vi "Open RS422A.vi"(4 "Source (\"\")":string, 6 "Timeout (25000)":u32=25000, 8 "error in (no error)":errorcluster, 10 "Address (1)":i32=1 min=1 max=99 step=1, 11 "VISA resource name":refnum<visa-resource-name>) -> (0 "error out":errorcluster, 3 "VISA resource name out":refnum<visa-resource-name>)   [LabVIEW 2020, in "Yokogawa GX Series.lvlib"]
doc: "Opens RS-422A/485."
uses:
  <instrlib>/Yokogawa GX Series/Yokogawa GX Series.lvlib
panel:
  # "msec"
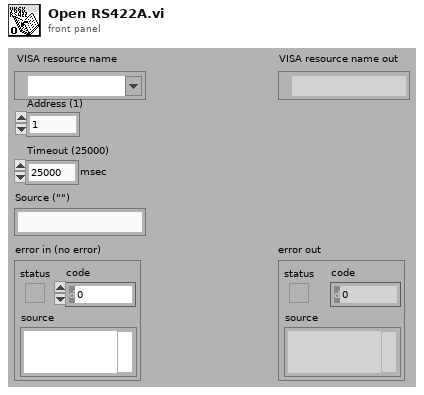
[diagram p1: front panel]
types:
  T1 = cluster{"User Name":string, "User ID":string, "Password":string, "Serial Auth Type (0: Not Auth)":u16, "SMARTDAC+ Type (0: Unknown)":u16, "Bluetooth Password":string}
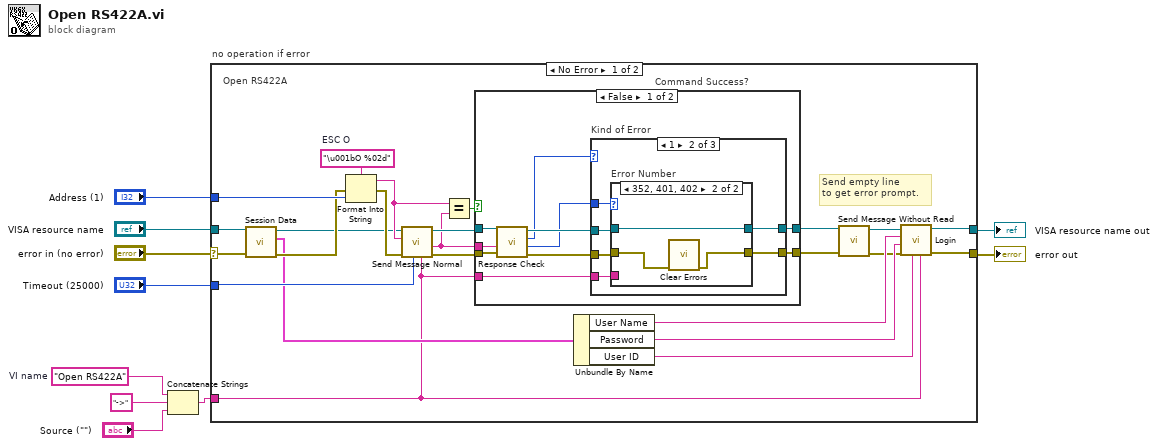
[diagram p0: block diagram]
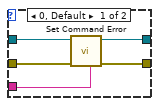
[diagram p3: hidden frame]
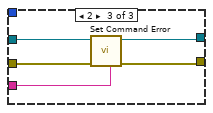
[diagram p4: hidden frame]
diagram:
  w4 = "Open RS422A"  # VI name
  n1 = Concatenate Strings(w4, "->", "Source (\"\")") -> (w2:string)
  n2 = case "no operation if error" shown="No Error" "error in (no error)" {
    selector: "error in (no error)" -> [w18 w68]
    tunnel: "Address (1)" -> [w34 _]
    tunnel: "VISA resource name" -> [w19 w69]
    tunnel: [w23 w69] -> w8
    tunnel: [w22 w68] -> w7
    tunnel: "Timeout (25000)" -> [w28 _]
    tunnel: w2 -> [w11 _]
    frame No Error {
      w33 = "\u001bO %02d"  # ESC O
      # "Send empty line\nto get error prompt."
      # "Open RS422A"
      n3 = call <instrlib>:"Session Data.vi"("error in (no error)"=w18, "VISA resource name"=w19) -> ("error out"=w17:errorcluster, "User Data Out"=w15:T1, "VISA resource name out"=w16:refnum<visa-resource-name>)  [unwired: 7 in]
      n4 = Format Into String(format string=w33, error in=w17, w34) -> (resulting string=w27:string, error out=w29:errorcluster)  [unwired: 1 in]
      n5 = call <instrlib>:"Send Message Normal.vi"("Source (\"\")"=w11, "Timeout (25000)"=w28, "error in (no error)"=w29, "Send Message (\"\")"=w27, "VISA resource name"=w16) -> ("error out"=w31:errorcluster, "Read Buffer"=w14:string, "VISA resource name out"=w30:refnum<visa-resource-name>)  [unwired: 4 out]
      n6 = Equal?(x=w27, y=w14) -> (x = y?=w32:bool)
      n7 = case "Command Success?" shown="False" w32 {
        tunnel: w30 -> [w41 w67]
        tunnel: [w44 w67] -> w21
        tunnel: w31 -> [w40 w66]
        tunnel: [w43 w66] -> w20
        tunnel: w11 -> [w42 _]
        tunnel: w14 -> [w39 _]
        frame False {
          n8 = call <instrlib>:"Response Check.vi"("error in (no error)"=w40, "Message In (\"\")"=w39, "VISA resource name"=w41) -> ("error out"=w37:errorcluster, "Internal Error Number"=w35:i32, "Response Type"=w36:i32, "VISA resource name out"=w38:refnum<visa-resource-name>)  [unwired: 4 in, 1 out]
          n9 = case "Kind of Error" shown="1" w36 {
            tunnel: [w46 w52 w63] -> w44
            tunnel: [w45 w51 w62] -> w43
            tunnel: w42 -> [_ w50 w61]
            tunnel: w38 -> [w46 w49 w65]
            tunnel: w37 -> [w45 w48 w64]
            tunnel: w35 -> [_ w47 _]
            frame 0, Default {
            }
            frame 1 {
              n10 = case "Error Number" shown="352, 401, 402" w47 {
                tunnel: w49 -> [w57 w60]
                tunnel: [w56 w60] -> w52
                tunnel: [w55 w59] -> w51
                tunnel: w48 -> [w54 w58]
                tunnel: w50 -> [w53 _]
                frame 0, Default {
                  n11 = call <instrlib>:"Set Command Error.vi"("Source (\"\")"=w53, "error in (no error)"=w54, "VISA resource name"=w57) -> ("error out"=w55:errorcluster, "VISA resource name out"=w56:refnum<visa-resource-name>)  [unwired: 7 out]
                }
                frame 352, 401, 402 {
                  n12 = call <vilib>:"Clear Errors.vi"("error in (no error)"=w58) -> ("error out"=w59:errorcluster)  [unwired: 5 in, 1 out]
                }
              }
            }
            frame 2 {
              n13 = call <instrlib>:"Set Command Error.vi"("Source (\"\")"=w61, "error in (no error)"=w64, "VISA resource name"=w65) -> ("error out"=w62:errorcluster, "VISA resource name out"=w63:refnum<visa-resource-name>)  [unwired: 7 out]
            }
          }
        }
        frame True {
        }
      }
      n14 = Unbundle By Name(w15) -> ("User Name"=w24:string, "Password"=w25:string, "User ID"=w26:string)
      n15 = call <instrlib>:"Send Message Without Read.vi"("error in (no error)"=w20, "VISA resource name"=w21) -> ("error out"=w12:errorcluster, "VISA resource name out"=w13:refnum<visa-resource-name>)  [unwired: 8 in]
      n16 = call <instrlib>:"Login.vi"("Source (\"\")"=w11, "User ID (\"\")"=w26, "error in (no error)"=w12, "Password (\"\")"=w25, "User Name (\"admin\")"=w24, "VISA resource name"=w13) -> ("error out"=w22:errorcluster, "VISA resource name out"=w23:refnum<visa-resource-name>)  [unwired: 4 in]
    }
    frame Error {
    }
  }
  "VISA resource name out" <- w8
  "error out" <- w7
